vi "Vision Thingie.vi"() -> (0 "z":dbl, 1 "z2":dbl)   [LabVIEW 2019]
uses:
  Robot Global Data.vi
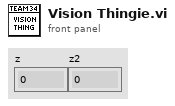
[diagram p1: front panel]
types:
  T1 = typedef "Vision Data.ctl" = cluster{"xOffset":dbl, "yOffset":dbl, "area":dbl, "skewOffset":dbl, "hasTarget":dbl}
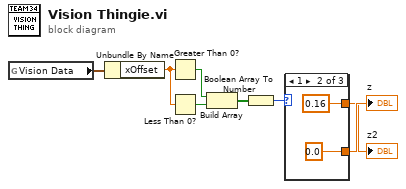
[diagram p0: block diagram]
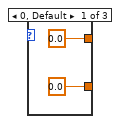
[diagram p2: hidden frame]
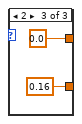
[diagram p3: hidden frame]
diagram:
  n1 = global read "Robot Global Data.vi" "Vision Data"() -> (w8:T1)
  n2 = Unbundle By Name(w8) -> ("xOffset"=w7:dbl)
  n3 = Greater Than 0?(x=w7) -> (x > 0?=w6:bool)
  n4 = Less Than 0?(x=w7) -> (x < 0?=w5:bool)
  n5 = Build Array(w6, w5) -> (w4:bool[])
  n6 = Boolean Array To Number(Boolean array=w4) -> (number=w3:u32)
  n7 = case shown="1" w3 {
    tunnel: [0.0 0.16 0.0] -> w1
    tunnel: [0.0 0.0 0.16] -> w2
    frame 0, Default {
    }
    frame 1 {
    }
    frame 2 {
    }
  }
  "z" <- w2
  "z2" <- w1
